vi "Vision Research Phantom Series PhCon PhNVMGetSaveRange.vi"(0 "CN in":u32=1, 5 "Error In (no error)":errorcluster) -> (14 "CN out":u32=1, 16 "pRng":T1, 19 "Error Out":errorcluster)   [LabVIEW 2013, in "VRI.lvlib"]
doc: "PhCon.dll\n\nPhNVMGetSaveRange\nHRESULT PhNVMGetSaveRange(UINT CN, PIMRANGE pRng);\n \nParameters Description\nCN (in) Camera number\npRng (in) Image range\nReturn HRESULT (0=Ok)\nComments Get the save range for the NVM Save or NVM \n continuous recording\n\nWritten by:\nBLOOMY CONTROLS, INC\nWINDSOR, CT 06095, USA\n860-298-9925\nwww.bloomy.com\nV1.0.0\nMay, 2004"
uses:
  VRI.lvlib
  _Type Defs/PHCon IMRANGE.ctl
  Phantom DLLs/PhCon.dll
panel:
  # "For instructions on the use of this VI, press Ctrl+H to display the help window and move the mouse over the icon, controls, and indicators"
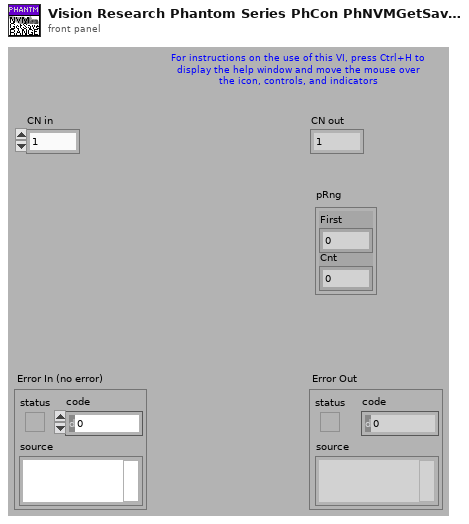
[diagram p1: front panel]
types:
  T1 = typedef "VRI.lvlib/PHCon IMRANGE.ctl" = cluster{"First":i32, "Cnt":u32}
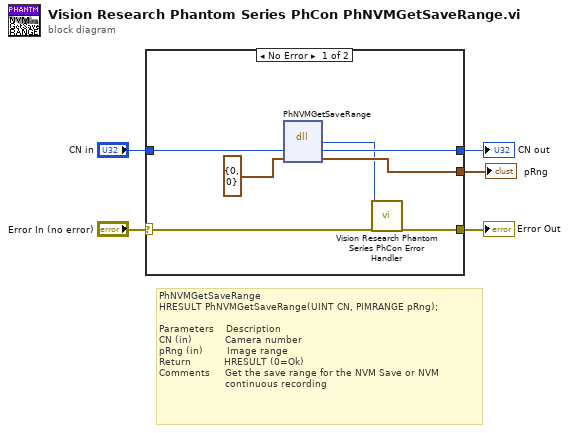
[diagram p0: block diagram]
diagram:
  # "PhNVMGetSaveRange\nHRESULT PhNVMGetSaveRange(UINT CN, PIMRANGE pRng);\n  \nParameters    Description\nCN (in)           Camera number\npRng (in)        Image range\nReturn           HRESULT (0=Ok)\nComments     Get the save range for the NVM Save or NVM \n                      continuous recording"
  n1 = case shown="No Error" "Error In (no error)" {
    selector: "Error In (no error)" -> [w12 w14]
    tunnel: [w11 w14] -> w4
    tunnel: "CN in" -> [w10 w13]
    tunnel: [w9 w13] -> w2
    tunnel: [w8 _] -> w1
    frame No Error {
      n2 = dll-call lib="C:/Projects/SDK/32-bit/Vision Research Phantom Series Labview Driver/Phantom DLLs/PhCon.dll" fn="PhNVMGetSaveRange"("CN"=w10, "pRng"=T1 {"First"=0, "Cnt"=0}) -> ("HRESULT"=w7:i32, "CN"=w9:u32, "pRng"=w8:T1)  [unwired: 3 in, 2 out]
      n3 = call "Vision Research Phantom Series PhCon Error Handler.vi"("ErrNo"=w7, "Error In (no error)"=w12) -> ("Error Out"=w11:errorcluster)  [unwired: 17 out]
    }
    frame Error {
    }
  }
  "Error Out" <- w4
  "CN out" <- w2
  "pRng" <- w1
